vi "test-new-clock-2.vi"() -> ()   [LabVIEW 2019]
uses:
  <vilib>/Utility/RT CPU Load.ctl
  <vilib>/NI_Real-Time Target Support.lvlib
panel:
  out "Loop5":i32
  out "Err Sum6":i32
  out "Clock6":dbl
  out "Err Sum5":i32
  out "Clock5":dbl
  out "CPU loads":T1[](array[typedef]) {"ISR (%)" format="%#.2f"; "Idle (%)" format="%#.2f"; "Background (%)" format="%#.2f"; "Normal (%)" format="%#.2f"; "Above Normal (%)" format="%#.2f"; "High (%)" format="%#.2g"; "Timed Structures (%)" format="%#.2g"; "Time Critical (%)" format="%#.2g"; "Total (%)" format="%#.2g"}
  out "Diff":dbl
  out "Err Sum4":i32
  out "Clock4":dbl
  out "Err Sum3":i32
  out "Clock3":dbl
  out "Err Sum2":i32
  out "Clock2":dbl
  out "Clock1":dbl
  out "Err Sum1":i32
  out "OS Clock":dbl format="%35.6f"
  out "Error Count":i32
  out "Loop Count":i32
  out "FPGA Clock":dbl format="%35.6f"
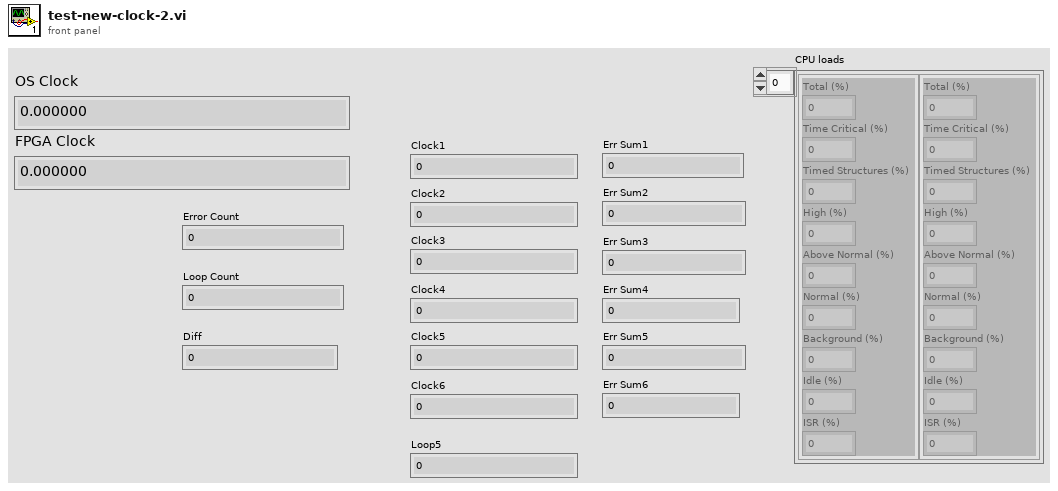
[diagram p1: front panel]
types:
  T1 = typedef "NI_Real-Time Target Support.lvlib/RT CPU Load.ctl" = cluster{"Total (%)":dbl, "Time Critical (%)":dbl, "Timed Structures (%)":dbl, "High (%)":dbl, "Above Normal (%)":dbl, "Normal (%)":dbl, "Background (%)":dbl, "Idle (%)":dbl, "ISR (%)":dbl}
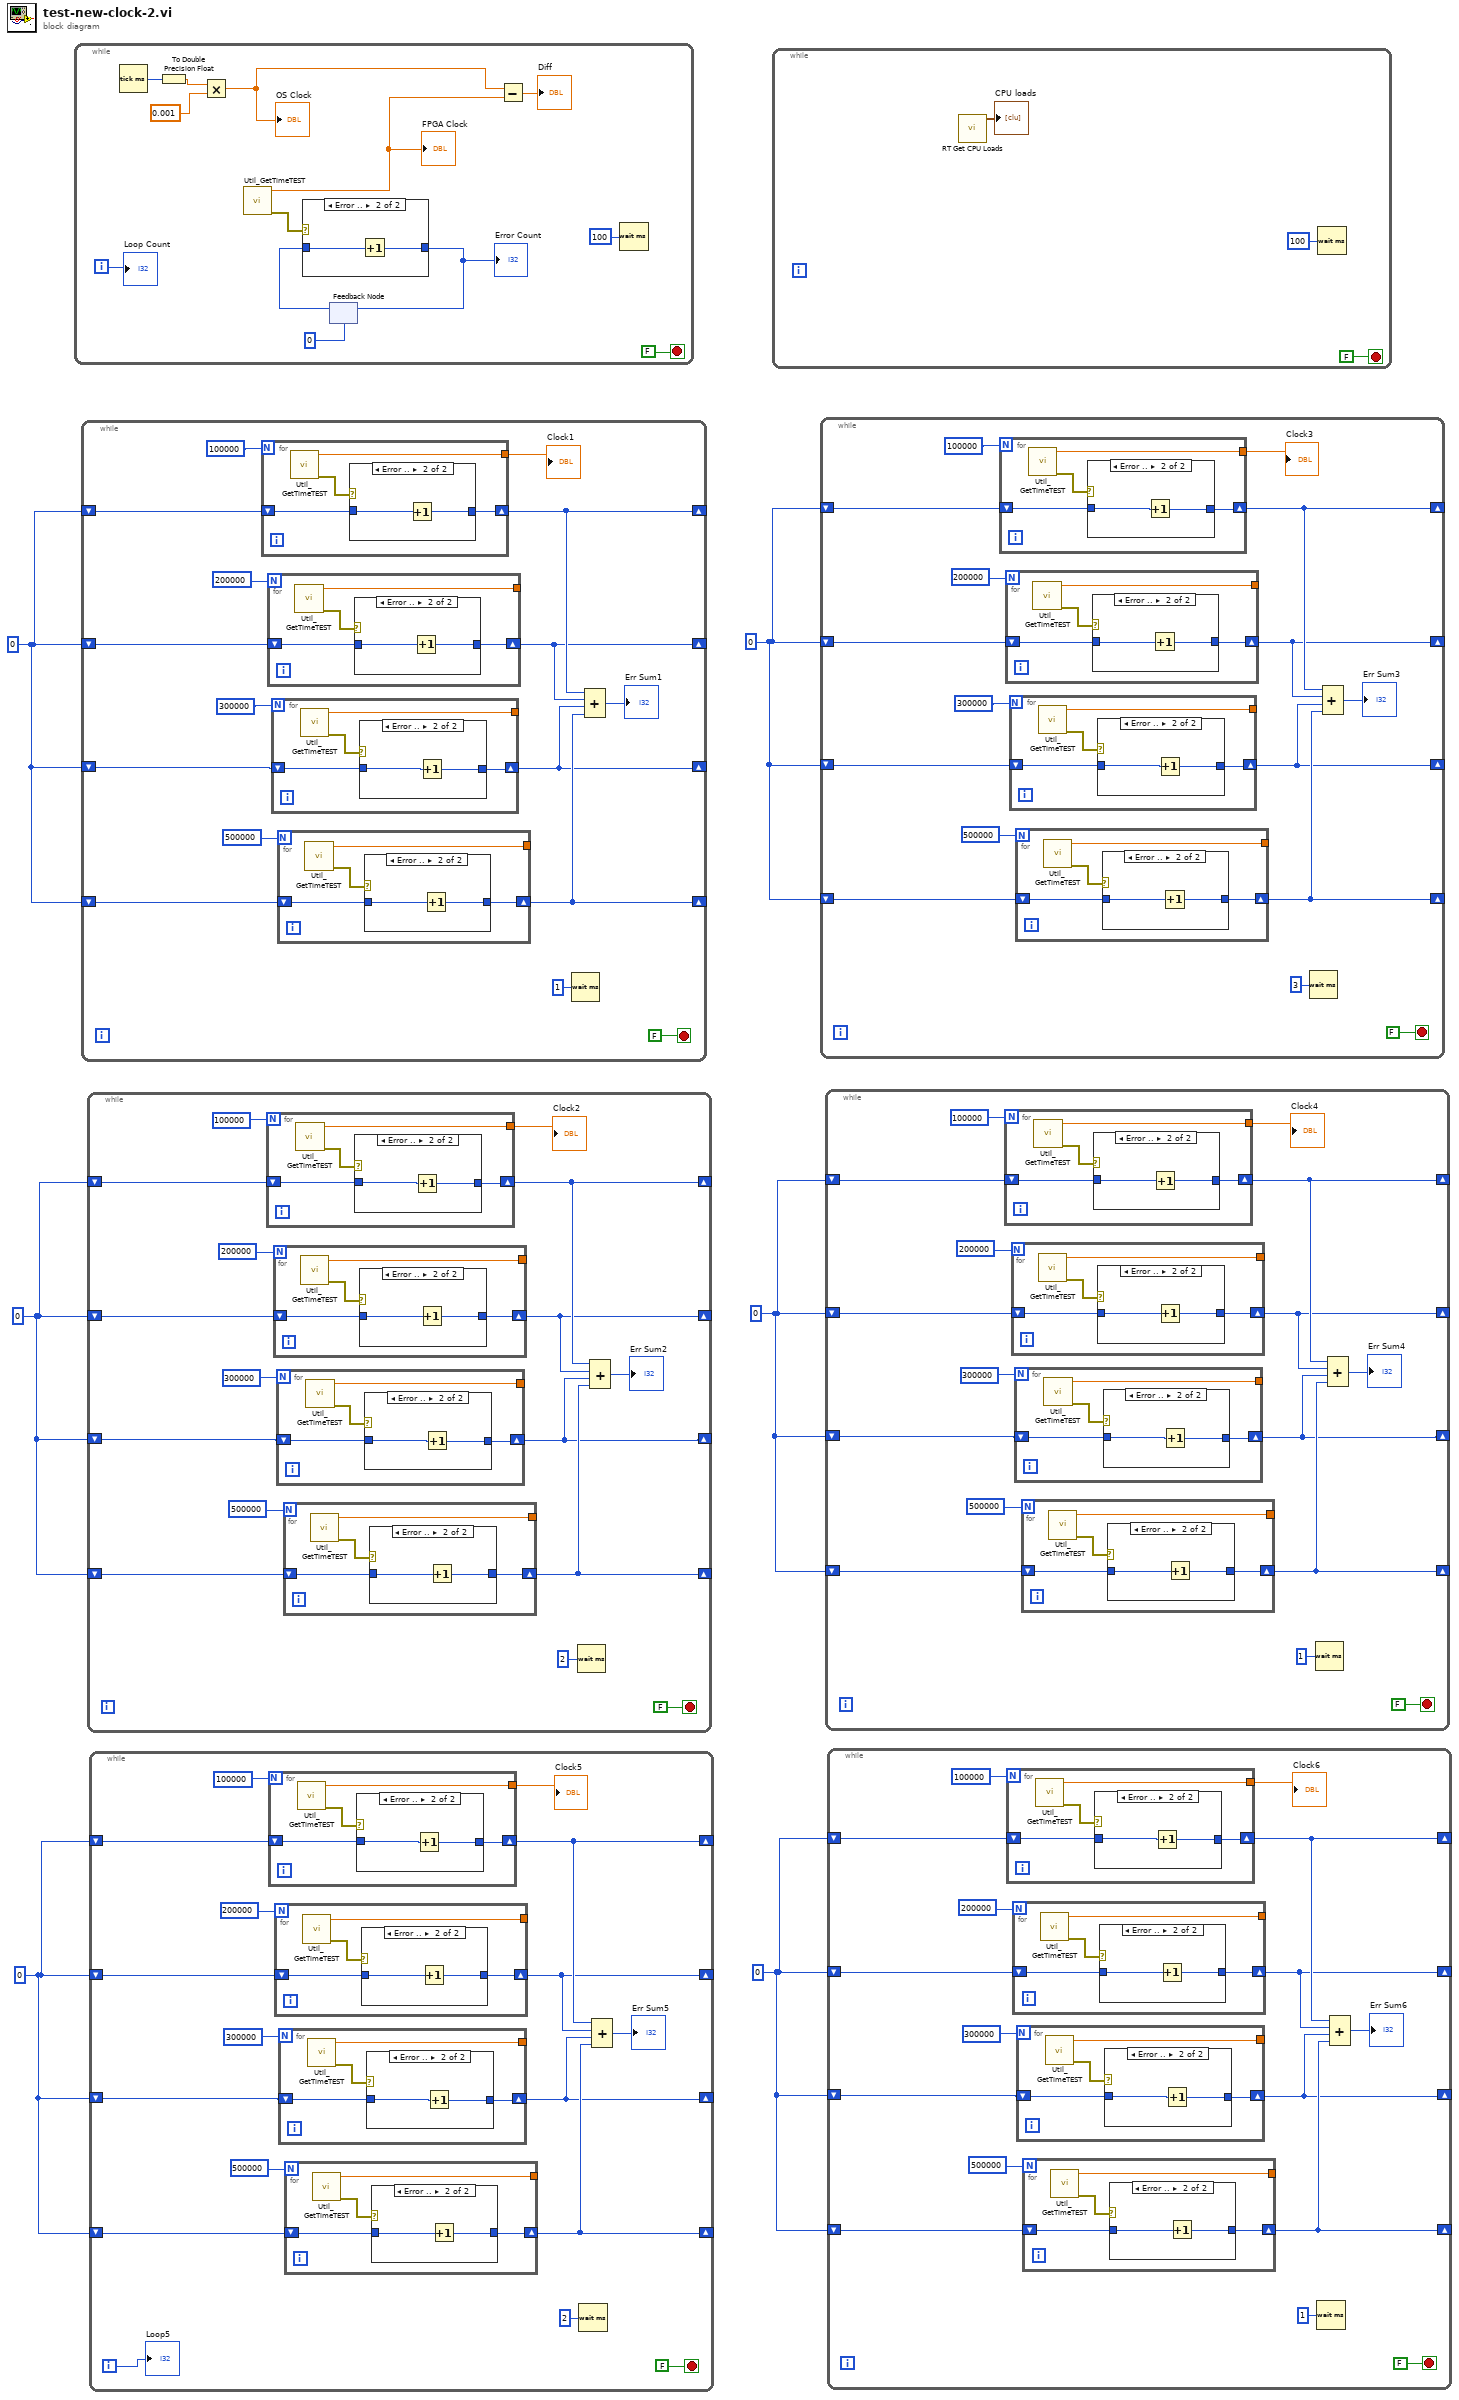
[diagram p0: block diagram]
diagram:
  w1 = 0
  w2 = 0
  w3 = 0
  w4 = 0
  w5 = 0
  w6 = 0
  n1 = while {
    i -> [w18]
    stop <- FALSE stop-if-true
    n2 = Tick Count (ms)() -> (millisecond timer value=w12:u32)
    n3 = To Double Precision Float(number=w12) -> (double precision float=w11:dbl)
    n4 = Multiply(x=w11, y=0.001) -> (x*y=w9:dbl)
    "OS Clock" <- w9
    n5 = call "Util_GetTimeTEST.vi"() -> ("error out"=w16:errorcluster, "FPGA_Time_Seconds"=w8:dbl)  [unwired: 10 in]
    "FPGA Clock" <- w8
    n6 = feedback #1(0) -> (w15:i32)
    n7 = case shown="Error .." w16 {
      tunnel: w15 -> [w20 w21]
      tunnel: [w20 w22] -> w14
      frame No Error {
      }
      frame Error {
        n8 = Increment(x=w21) -> (x+1=w22:i32)
      }
    }
    "Error Count" <- w14
    n9 = feedback-in #1(w14) -> ()
    n10 = Subtract(x=w9, y=w8) -> (x-y=→"Diff":dbl)
    n11 = Wait (ms)(milliseconds to wait=u32 100) -> ()  [unwired: 1 out]
    "Loop Count" <- w18
  }
  n12 = while {
    shift-right: [w27] -> _
    shift-left: w6 -> [w34]
    shift-right: [w28] -> _
    shift-left: w6 -> [w33]
    shift-right: [w25] -> _
    shift-left: w6 -> [w30]
    shift-right: [w26] -> _
    shift-left: w6 -> [w29]
    stop <- FALSE stop-if-true
    n13 = for {
      N: 100000 -> [_]
      shift-right: [w61] -> w28
      shift-left: w33 -> [w62]
      tunnel: [w60] -> w23
      n14 = call "Util_GetTimeTEST.vi"() -> ("error out"=w63:errorcluster, "FPGA_Time_Seconds"=w60:dbl)  [unwired: 10 in]
      n15 = case shown="Error .." w63 {
        tunnel: [w64 w66] -> w61
        tunnel: w62 -> [w64 w65]
        frame No Error {
        }
        frame Error {
          n16 = Increment(x=w65) -> (x+1=w66:i32)
        }
      }
    }
    "Clock1" <- w23
    n17 = for {
      N: 200000 -> [_]
      shift-right: [w54] -> w27
      shift-left: w34 -> [w55]
      tunnel: [w53] -> _
      n18 = call "Util_GetTimeTEST.vi"() -> ("error out"=w56:errorcluster, "FPGA_Time_Seconds"=w53:dbl)  [unwired: 10 in]
      n19 = case shown="Error .." w56 {
        tunnel: [w57 w59] -> w54
        tunnel: w55 -> [w57 w58]
        frame No Error {
        }
        frame Error {
          n20 = Increment(x=w58) -> (x+1=w59:i32)
        }
      }
    }
    n21 = for {
      N: 300000 -> [_]
      shift-right: [w47] -> w25
      shift-left: w30 -> [w48]
      tunnel: [w46] -> _
      n22 = call "Util_GetTimeTEST.vi"() -> ("error out"=w49:errorcluster, "FPGA_Time_Seconds"=w46:dbl)  [unwired: 10 in]
      n23 = case shown="Error .." w49 {
        tunnel: [w50 w52] -> w47
        tunnel: w48 -> [w50 w51]
        frame No Error {
        }
        frame Error {
          n24 = Increment(x=w51) -> (x+1=w52:i32)
        }
      }
    }
    n25 = for {
      N: 500000 -> [_]
      shift-right: [w40] -> w26
      shift-left: w29 -> [w41]
      tunnel: [w39] -> _
      n26 = call "Util_GetTimeTEST.vi"() -> ("error out"=w42:errorcluster, "FPGA_Time_Seconds"=w39:dbl)  [unwired: 10 in]
      n27 = case shown="Error .." w42 {
        tunnel: [w43 w45] -> w40
        tunnel: w41 -> [w43 w44]
        frame No Error {
        }
        frame Error {
          n28 = Increment(x=w44) -> (x+1=w45:i32)
        }
      }
    }
    n29 = Wait (ms)(milliseconds to wait=u32 1) -> ()  [unwired: 1 out]
    n30 = Compound Arithmetic op=ADD(w28, w27, w25, w26) -> (→"Err Sum1":i32)
  }
  n31 = while {
    shift-right: [w71] -> _
    shift-left: w5 -> [w78]
    shift-right: [w72] -> _
    shift-left: w5 -> [w77]
    shift-right: [w69] -> _
    shift-left: w5 -> [w74]
    shift-right: [w70] -> _
    shift-left: w5 -> [w73]
    stop <- FALSE stop-if-true
    n32 = for {
      N: 100000 -> [_]
      shift-right: [w105] -> w72
      shift-left: w77 -> [w106]
      tunnel: [w104] -> w67
      n33 = call "Util_GetTimeTEST.vi"() -> ("error out"=w107:errorcluster, "FPGA_Time_Seconds"=w104:dbl)  [unwired: 10 in]
      n34 = case shown="Error .." w107 {
        tunnel: [w108 w110] -> w105
        tunnel: w106 -> [w108 w109]
        frame No Error {
        }
        frame Error {
          n35 = Increment(x=w109) -> (x+1=w110:i32)
        }
      }
    }
    "Clock2" <- w67
    n36 = for {
      N: 200000 -> [_]
      shift-right: [w98] -> w71
      shift-left: w78 -> [w99]
      tunnel: [w97] -> _
      n37 = call "Util_GetTimeTEST.vi"() -> ("error out"=w100:errorcluster, "FPGA_Time_Seconds"=w97:dbl)  [unwired: 10 in]
      n38 = case shown="Error .." w100 {
        tunnel: [w101 w103] -> w98
        tunnel: w99 -> [w101 w102]
        frame No Error {
        }
        frame Error {
          n39 = Increment(x=w102) -> (x+1=w103:i32)
        }
      }
    }
    n40 = for {
      N: 300000 -> [_]
      shift-right: [w91] -> w69
      shift-left: w74 -> [w92]
      tunnel: [w90] -> _
      n41 = call "Util_GetTimeTEST.vi"() -> ("error out"=w93:errorcluster, "FPGA_Time_Seconds"=w90:dbl)  [unwired: 10 in]
      n42 = case shown="Error .." w93 {
        tunnel: [w94 w96] -> w91
        tunnel: w92 -> [w94 w95]
        frame No Error {
        }
        frame Error {
          n43 = Increment(x=w95) -> (x+1=w96:i32)
        }
      }
    }
    n44 = for {
      N: 500000 -> [_]
      shift-right: [w84] -> w70
      shift-left: w73 -> [w85]
      tunnel: [w83] -> _
      n45 = call "Util_GetTimeTEST.vi"() -> ("error out"=w86:errorcluster, "FPGA_Time_Seconds"=w83:dbl)  [unwired: 10 in]
      n46 = case shown="Error .." w86 {
        tunnel: [w87 w89] -> w84
        tunnel: w85 -> [w87 w88]
        frame No Error {
        }
        frame Error {
          n47 = Increment(x=w88) -> (x+1=w89:i32)
        }
      }
    }
    n48 = Wait (ms)(milliseconds to wait=u32 2) -> ()  [unwired: 1 out]
    n49 = Compound Arithmetic op=ADD(w72, w71, w69, w70) -> (→"Err Sum2":i32)
  }
  n50 = while {
    shift-right: [w116] -> _
    shift-left: w2 -> [w123]
    shift-right: [w117] -> _
    shift-left: w2 -> [w122]
    shift-right: [w114] -> _
    shift-left: w2 -> [w119]
    shift-right: [w115] -> _
    shift-left: w2 -> [w118]
    i -> [w111]
    stop <- FALSE stop-if-true
    n51 = for {
      N: 100000 -> [_]
      shift-right: [w150] -> w117
      shift-left: w122 -> [w151]
      tunnel: [w149] -> w112
      n52 = call "Util_GetTimeTEST.vi"() -> ("error out"=w152:errorcluster, "FPGA_Time_Seconds"=w149:dbl)  [unwired: 10 in]
      n53 = case shown="Error .." w152 {
        tunnel: [w153 w155] -> w150
        tunnel: w151 -> [w153 w154]
        frame No Error {
        }
        frame Error {
          n54 = Increment(x=w154) -> (x+1=w155:i32)
        }
      }
    }
    "Clock5" <- w112
    n55 = for {
      N: 200000 -> [_]
      shift-right: [w143] -> w116
      shift-left: w123 -> [w144]
      tunnel: [w142] -> _
      n56 = call "Util_GetTimeTEST.vi"() -> ("error out"=w145:errorcluster, "FPGA_Time_Seconds"=w142:dbl)  [unwired: 10 in]
      n57 = case shown="Error .." w145 {
        tunnel: [w146 w148] -> w143
        tunnel: w144 -> [w146 w147]
        frame No Error {
        }
        frame Error {
          n58 = Increment(x=w147) -> (x+1=w148:i32)
        }
      }
    }
    n59 = for {
      N: 300000 -> [_]
      shift-right: [w136] -> w114
      shift-left: w119 -> [w137]
      tunnel: [w135] -> _
      n60 = call "Util_GetTimeTEST.vi"() -> ("error out"=w138:errorcluster, "FPGA_Time_Seconds"=w135:dbl)  [unwired: 10 in]
      n61 = case shown="Error .." w138 {
        tunnel: [w139 w141] -> w136
        tunnel: w137 -> [w139 w140]
        frame No Error {
        }
        frame Error {
          n62 = Increment(x=w140) -> (x+1=w141:i32)
        }
      }
    }
    n63 = for {
      N: 500000 -> [_]
      shift-right: [w129] -> w115
      shift-left: w118 -> [w130]
      tunnel: [w128] -> _
      n64 = call "Util_GetTimeTEST.vi"() -> ("error out"=w131:errorcluster, "FPGA_Time_Seconds"=w128:dbl)  [unwired: 10 in]
      n65 = case shown="Error .." w131 {
        tunnel: [w132 w134] -> w129
        tunnel: w130 -> [w132 w133]
        frame No Error {
        }
        frame Error {
          n66 = Increment(x=w133) -> (x+1=w134:i32)
        }
      }
    }
    n67 = Wait (ms)(milliseconds to wait=u32 2) -> ()  [unwired: 1 out]
    n68 = Compound Arithmetic op=ADD(w117, w116, w114, w115) -> (→"Err Sum5":i32)
    "Loop5" <- w111
  }
  n69 = while {
    stop <- FALSE stop-if-true
    n70 = call <vilib>:"RT Get CPU Loads.vi"() -> ("CPU loads"=→"CPU loads":T1[])  [unwired: 10 in, 1 out]
    n71 = Wait (ms)(milliseconds to wait=u32 100) -> ()  [unwired: 1 out]
  }
  n72 = while {
    shift-right: [w163] -> _
    shift-left: w4 -> [w170]
    shift-right: [w164] -> _
    shift-left: w4 -> [w169]
    shift-right: [w161] -> _
    shift-left: w4 -> [w166]
    shift-right: [w162] -> _
    shift-left: w4 -> [w165]
    stop <- FALSE stop-if-true
    n73 = for {
      N: 100000 -> [_]
      shift-right: [w197] -> w164
      shift-left: w169 -> [w198]
      tunnel: [w196] -> w159
      n74 = call "Util_GetTimeTEST.vi"() -> ("error out"=w199:errorcluster, "FPGA_Time_Seconds"=w196:dbl)  [unwired: 10 in]
      n75 = case shown="Error .." w199 {
        tunnel: [w200 w202] -> w197
        tunnel: w198 -> [w200 w201]
        frame No Error {
        }
        frame Error {
          n76 = Increment(x=w201) -> (x+1=w202:i32)
        }
      }
    }
    "Clock3" <- w159
    n77 = for {
      N: 200000 -> [_]
      shift-right: [w190] -> w163
      shift-left: w170 -> [w191]
      tunnel: [w189] -> _
      n78 = call "Util_GetTimeTEST.vi"() -> ("error out"=w192:errorcluster, "FPGA_Time_Seconds"=w189:dbl)  [unwired: 10 in]
      n79 = case shown="Error .." w192 {
        tunnel: [w193 w195] -> w190
        tunnel: w191 -> [w193 w194]
        frame No Error {
        }
        frame Error {
          n80 = Increment(x=w194) -> (x+1=w195:i32)
        }
      }
    }
    n81 = for {
      N: 300000 -> [_]
      shift-right: [w183] -> w161
      shift-left: w166 -> [w184]
      tunnel: [w182] -> _
      n82 = call "Util_GetTimeTEST.vi"() -> ("error out"=w185:errorcluster, "FPGA_Time_Seconds"=w182:dbl)  [unwired: 10 in]
      n83 = case shown="Error .." w185 {
        tunnel: [w186 w188] -> w183
        tunnel: w184 -> [w186 w187]
        frame No Error {
        }
        frame Error {
          n84 = Increment(x=w187) -> (x+1=w188:i32)
        }
      }
    }
    n85 = for {
      N: 500000 -> [_]
      shift-right: [w176] -> w162
      shift-left: w165 -> [w177]
      tunnel: [w175] -> _
      n86 = call "Util_GetTimeTEST.vi"() -> ("error out"=w178:errorcluster, "FPGA_Time_Seconds"=w175:dbl)  [unwired: 10 in]
      n87 = case shown="Error .." w178 {
        tunnel: [w179 w181] -> w176
        tunnel: w177 -> [w179 w180]
        frame No Error {
        }
        frame Error {
          n88 = Increment(x=w180) -> (x+1=w181:i32)
        }
      }
    }
    n89 = Wait (ms)(milliseconds to wait=u32 3) -> ()  [unwired: 1 out]
    n90 = Compound Arithmetic op=ADD(w164, w163, w161, w162) -> (→"Err Sum3":i32)
  }
  n91 = while {
    shift-right: [w207] -> _
    shift-left: w3 -> [w214]
    shift-right: [w208] -> _
    shift-left: w3 -> [w213]
    shift-right: [w205] -> _
    shift-left: w3 -> [w210]
    shift-right: [w206] -> _
    shift-left: w3 -> [w209]
    stop <- FALSE stop-if-true
    n92 = for {
      N: 100000 -> [_]
      shift-right: [w241] -> w208
      shift-left: w213 -> [w242]
      tunnel: [w240] -> w203
      n93 = call "Util_GetTimeTEST.vi"() -> ("error out"=w243:errorcluster, "FPGA_Time_Seconds"=w240:dbl)  [unwired: 10 in]
      n94 = case shown="Error .." w243 {
        tunnel: [w244 w246] -> w241
        tunnel: w242 -> [w244 w245]
        frame No Error {
        }
        frame Error {
          n95 = Increment(x=w245) -> (x+1=w246:i32)
        }
      }
    }
    "Clock4" <- w203
    n96 = for {
      N: 200000 -> [_]
      shift-right: [w234] -> w207
      shift-left: w214 -> [w235]
      tunnel: [w233] -> _
      n97 = call "Util_GetTimeTEST.vi"() -> ("error out"=w236:errorcluster, "FPGA_Time_Seconds"=w233:dbl)  [unwired: 10 in]
      n98 = case shown="Error .." w236 {
        tunnel: [w237 w239] -> w234
        tunnel: w235 -> [w237 w238]
        frame No Error {
        }
        frame Error {
          n99 = Increment(x=w238) -> (x+1=w239:i32)
        }
      }
    }
    n100 = for {
      N: 300000 -> [_]
      shift-right: [w227] -> w205
      shift-left: w210 -> [w228]
      tunnel: [w226] -> _
      n101 = call "Util_GetTimeTEST.vi"() -> ("error out"=w229:errorcluster, "FPGA_Time_Seconds"=w226:dbl)  [unwired: 10 in]
      n102 = case shown="Error .." w229 {
        tunnel: [w230 w232] -> w227
        tunnel: w228 -> [w230 w231]
        frame No Error {
        }
        frame Error {
          n103 = Increment(x=w231) -> (x+1=w232:i32)
        }
      }
    }
    n104 = for {
      N: 500000 -> [_]
      shift-right: [w220] -> w206
      shift-left: w209 -> [w221]
      tunnel: [w219] -> _
      n105 = call "Util_GetTimeTEST.vi"() -> ("error out"=w222:errorcluster, "FPGA_Time_Seconds"=w219:dbl)  [unwired: 10 in]
      n106 = case shown="Error .." w222 {
        tunnel: [w223 w225] -> w220
        tunnel: w221 -> [w223 w224]
        frame No Error {
        }
        frame Error {
          n107 = Increment(x=w224) -> (x+1=w225:i32)
        }
      }
    }
    n108 = Wait (ms)(milliseconds to wait=u32 1) -> ()  [unwired: 1 out]
    n109 = Compound Arithmetic op=ADD(w208, w207, w205, w206) -> (→"Err Sum4":i32)
  }
  n110 = while {
    shift-right: [w251] -> _
    shift-left: w1 -> [w258]
    shift-right: [w252] -> _
    shift-left: w1 -> [w257]
    shift-right: [w249] -> _
    shift-left: w1 -> [w254]
    shift-right: [w250] -> _
    shift-left: w1 -> [w253]
    stop <- FALSE stop-if-true
    n111 = for {
      N: 100000 -> [_]
      shift-right: [w285] -> w252
      shift-left: w257 -> [w286]
      tunnel: [w284] -> w247
      n112 = call "Util_GetTimeTEST.vi"() -> ("error out"=w287:errorcluster, "FPGA_Time_Seconds"=w284:dbl)  [unwired: 10 in]
      n113 = case shown="Error .." w287 {
        tunnel: [w288 w290] -> w285
        tunnel: w286 -> [w288 w289]
        frame No Error {
        }
        frame Error {
          n114 = Increment(x=w289) -> (x+1=w290:i32)
        }
      }
    }
    "Clock6" <- w247
    n115 = for {
      N: 200000 -> [_]
      shift-right: [w278] -> w251
      shift-left: w258 -> [w279]
      tunnel: [w277] -> _
      n116 = call "Util_GetTimeTEST.vi"() -> ("error out"=w280:errorcluster, "FPGA_Time_Seconds"=w277:dbl)  [unwired: 10 in]
      n117 = case shown="Error .." w280 {
        tunnel: [w281 w283] -> w278
        tunnel: w279 -> [w281 w282]
        frame No Error {
        }
        frame Error {
          n118 = Increment(x=w282) -> (x+1=w283:i32)
        }
      }
    }
    n119 = for {
      N: 300000 -> [_]
      shift-right: [w271] -> w249
      shift-left: w254 -> [w272]
      tunnel: [w270] -> _
      n120 = call "Util_GetTimeTEST.vi"() -> ("error out"=w273:errorcluster, "FPGA_Time_Seconds"=w270:dbl)  [unwired: 10 in]
      n121 = case shown="Error .." w273 {
        tunnel: [w274 w276] -> w271
        tunnel: w272 -> [w274 w275]
        frame No Error {
        }
        frame Error {
          n122 = Increment(x=w275) -> (x+1=w276:i32)
        }
      }
    }
    n123 = for {
      N: 500000 -> [_]
      shift-right: [w264] -> w250
      shift-left: w253 -> [w265]
      tunnel: [w263] -> _
      n124 = call "Util_GetTimeTEST.vi"() -> ("error out"=w266:errorcluster, "FPGA_Time_Seconds"=w263:dbl)  [unwired: 10 in]
      n125 = case shown="Error .." w266 {
        tunnel: [w267 w269] -> w264
        tunnel: w265 -> [w267 w268]
        frame No Error {
        }
        frame Error {
          n126 = Increment(x=w268) -> (x+1=w269:i32)
        }
      }
    }
    n127 = Wait (ms)(milliseconds to wait=u32 1) -> ()  [unwired: 1 out]
    n128 = Compound Arithmetic op=ADD(w252, w251, w249, w250) -> (→"Err Sum6":i32)
  }
